vi "Add Floor Lines to Grid.vi"(11 "Grig in":T1[][](array[typedef])=[[enum."Air", enum."Air", enum."Air", enum."Air", enum."Air", enum."Air", enum."Start", enum."Air", enum."Air", enum."Air"], [enum."Air", enum."Air", enum."Air", enum."Air", enum."Air", enum."Air", enum."Air", enum."Air", enum."Air", enum."Air"], [enum."Air", enum."Air", enum."Air", enum."Air", enum."Air", enum."Air", enum."Air", enum."Air", enum."Air", enum."Air"], [enum."Air", enum."Air", enum."Air", enum."Air", enum."Air", enum."Air", enum."Air", enum."Air", enum."Air", enum."Air"], [enum."Air", enum."Air", enum."Air", enum."Air", enum."Rock", enum."Air", enum."Air", enum."Air", enum."Rock", enum."Rock"], [enum."Air", enum."Air", enum."Air", enum."Air", enum."Rock", enum."Air", enum."Air", enum."Air", enum."Rock", enum."Air"], [enum."Air", enum."Air", enum."Rock", enum."Rock", enum."Rock", enum."Air", enum."Air", enum."Air", enum."Rock", enum."Air"], [enum."Air", enum."Air", enum."Air", enum."Air", enum."Air", enum."Air", enum."Air", enum."Air", enum."Rock", enum."Air"], [enum."Air", enum."Air", enum."Air", enum."Air", enum."Air", enum."Air", enum."Air", enum."Air", enum."Rock", enum."Air"], [enum."Rock", enum."Rock", enum."Rock", enum."Rock", enum."Rock", enum."Rock", enum."Rock", enum."Rock", enum."Rock", enum."Air"]]) -> (3 "output array":T1[][](array[typedef]))   [LabVIEW 2020]
uses:
  RB ENUM_Space ID.ctl
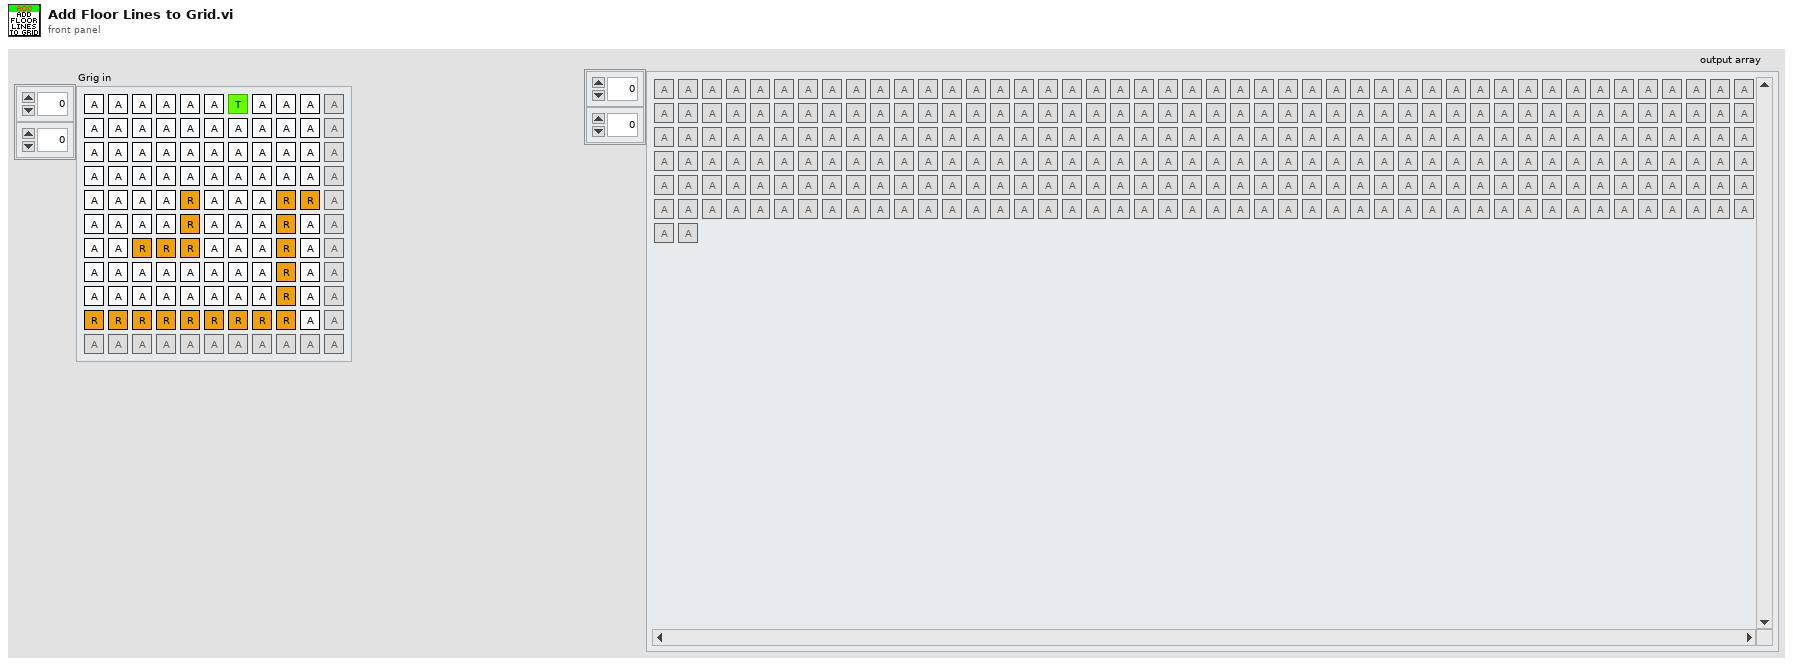
[diagram p1: front panel]
types:
  T1 = typedef "RB ENUM_Space ID.ctl" = enum32{"Air", "Sand", "Rock", "Start", "Abyss"}
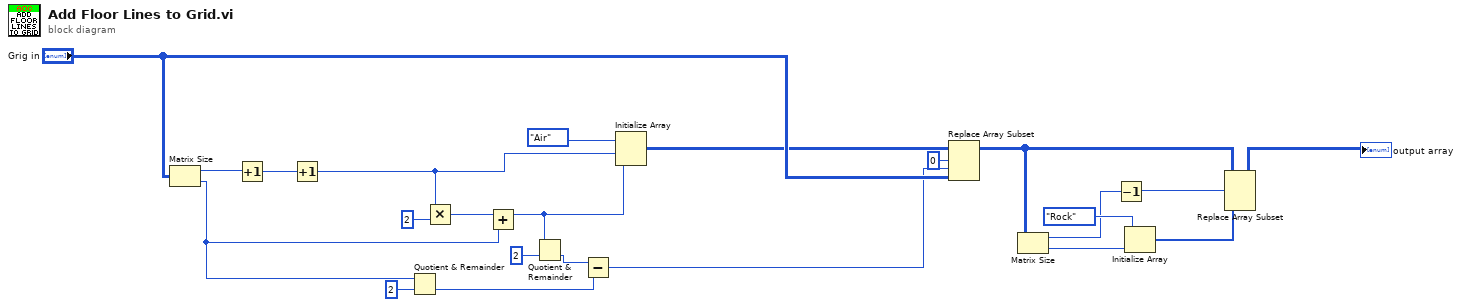
[diagram p0: block diagram]
diagram:
  n1 = Matrix Size(0:"Grig in") -> (1:w23:i32, 2:w8:i32)
  n2 = Increment(x=w23) -> (x+1=w22:i32)
  n3 = Increment(x=w22) -> (x+1=w9:i32)
  n4 = Quotient & Remainder(x=w8, y=2) -> (floor(x/y)=w12:i32)  [unwired: 1 out]
  n5 = Multiply(x=w9, y=2) -> (x*y=w19:i32)
  n6 = Add(x=w19, y=w8) -> (x+y=w18:i32)
  n7 = Quotient & Remainder(x=w18, y=2) -> (floor(x/y)=w14:i32)  [unwired: 1 out]
  n8 = Subtract(x=w14, y=w12) -> (x-y=w11:i32)
  n9 = Initialize Array(RB_ENUM_Space_ID."Air" ("Space"), w9, w18) -> (w10:T1[][])
  n10 = Replace Array Subset(array=w10, new element="Grig in", index (row)=0, index (col)=w11) -> (w5:T1[][])
  n11 = Matrix Size(0:w5) -> (1:w2:i32, 2:w7:i32)
  n12 = Decrement(x=w2) -> (x-1=w1:i32)
  n13 = Initialize Array(RB_ENUM_Space_ID."Rock" ("Space"), w7) -> (w3:T1[])
  n14 = Replace Array Subset(array=w5, new element=w3, index (row)=w1) -> (→"output array":T1[][])  [unwired: 1 in]
